vi "Enum Selected Value.vi"(8 "error in":errorcluster, 11 "Enum":refnum<vi>) -> (0 "error out":errorcluster, 1 "Value":i32, 2 "Value":string)   [LabVIEW 2013, in "Table Manager.lvlib"]
uses:
  Table Manager.lvlib
  <vilib>/NI/Tag Bus/tag/Data Type.ctl
  <vilib>/NI/Tag Bus/tag/tag descriptor.lvclass
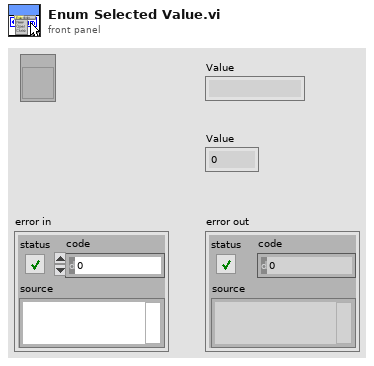
[diagram p1: front panel]
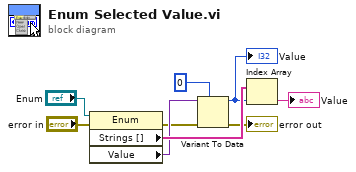
[diagram p0: block diagram]
diagram:
  n1 = property class="Enum"(reference="Enum", error in="error in") -> (error out=w2:errorcluster, "Strings []"=w9:string[], "Value"=w5:variant)  [unwired: 1 out]
  n2 = Variant To Data(error in=w2, type=0, Variant=w5) -> (data=w4:i32, error out=→"error out":errorcluster)
  "Value" <- w4
  n3 = Index Array(array=w9, index=w4) -> (element=→"Value":string)
